vi "basic_subvi_plotPNG_v2_170407.vi"(6 "Plot and Save Options":T2={"Color"=[0, 16711680, 6618880, 16860, 16750610, 4390878, 8388847, 16775234, 5878015, 16740807], "X axis label"="example x", "Y axis label"="example y", "BG color"=16776176, "% axis off"=0.1, "% margin "=2.0, "F: JPEG\nT: PNG"=TRUE, "Font"={"Font Name"="Times New Roman", "Size"=20, "Bold"=TRUE, "Italic"=FALSE, "Underline"=FALSE, "Strikeout"=FALSE, "Color"=0}, "Plot Line Width"=2, "X format str"="%.2f", "Y format str"="%.2f", "axis range"={"Max X scale"=0.0, "Min X scale"=0.0, "Max Y scale"=0.0, "Min Y scale"=0.0}, "auto scale?"=TRUE}, 8 "Path":path, 9 "Graph ref in":refnum<vi>) -> (4 "Graph (ploted) ref out":refnum<vi>)   [LabVIEW 2020, in "BasicVIs.lvlib"]
uses:
  BasicVIs.lvlib
  <vilib>/Utility/miscctls.llb/LVFontTypeDef.ctl
panel:
  out "Graph ref in valid?":bool
  out "path out":path
  out "error out":errorcluster
  in  "error in (no error)":errorcluster
  out "Graph":cluster{dbl[], dbl[]}[](graph)=[{[0.0, 1.0, 1.0, 0.0, 0.0], [0.0, 0.0, 1.0, 1.0, 0.0]}]
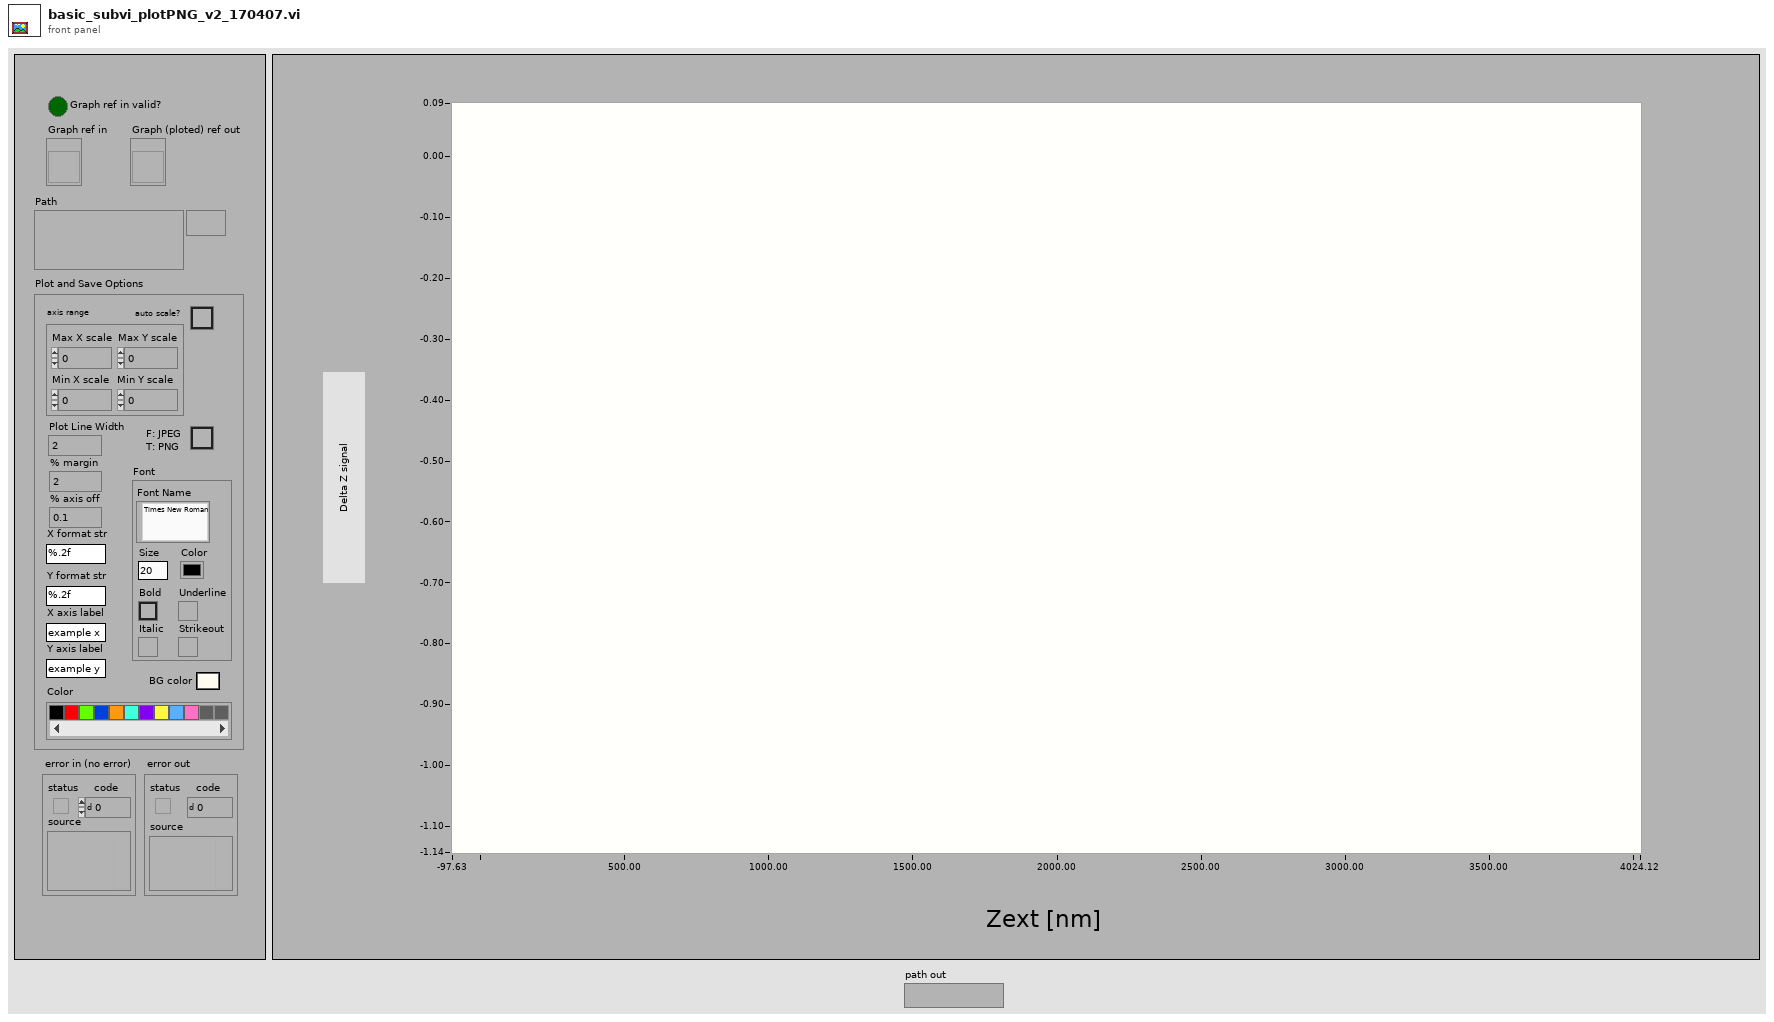
[diagram p1: front panel]
types:
  T1 = typedef "LVFontTypeDef.ctl" = cluster{"Font Name":string, "Size":u16, "Bold":bool, "Italic":bool, "Underline":bool, "Strikeout":bool, "Color":u32}
  T2 = cluster{"Color":u32[], "X axis label":string, "Y axis label":string, "BG color":u32, "% axis off":dbl, "% margin ":dbl, "F: JPEG\nT: PNG":bool, "Font":T1, "Plot Line Width":u8, "X format str":string, "Y format str":string, "axis range":cluster{"Max X scale":dbl, "Min X scale":dbl, "Max Y scale":dbl, "Min Y scale":dbl}, "auto scale?":bool}
  T3 = cluster{"Max X scale":dbl, "Min X scale":dbl, "Max Y scale":dbl, "Min Y scale":dbl}
  T4 = typedef "imagedata.ctl" = cluster{"image type":i32, "image depth":i32, "image":u8[], "mask":u8[], "colors":u32[], "Rectangle":cluster{"left":i16, "top":i16, "right":i16, "bottom":i16}}
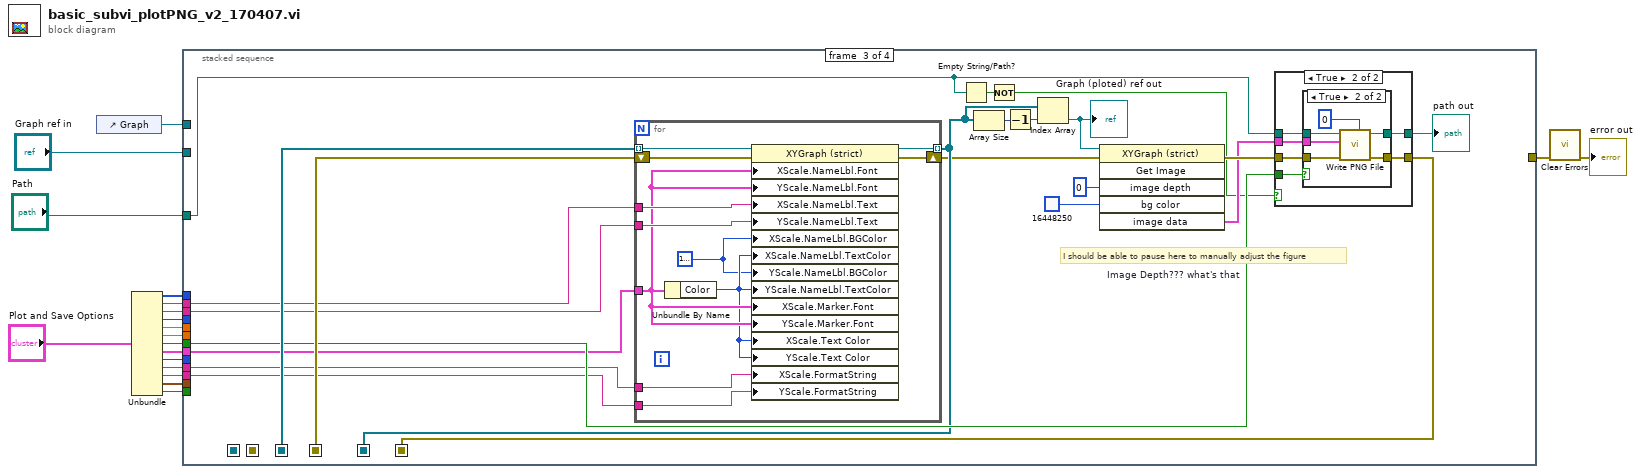
[diagram p0: block diagram]
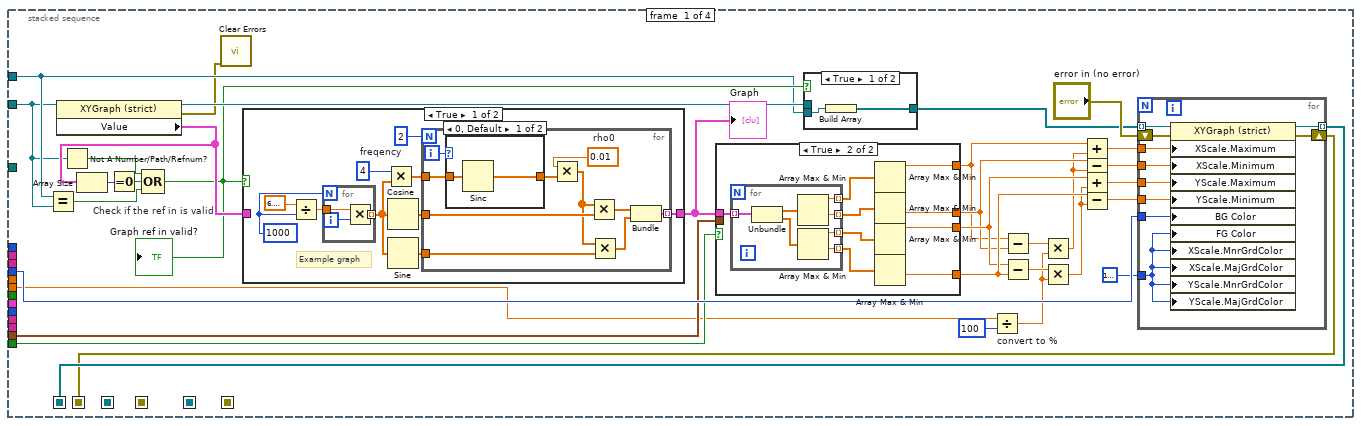
[diagram p2: hidden frame]
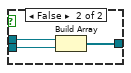
[diagram p3: hidden frame]
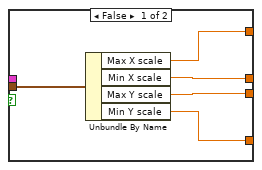
[diagram p4: hidden frame]
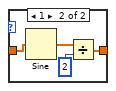
[diagram p5: hidden frame]
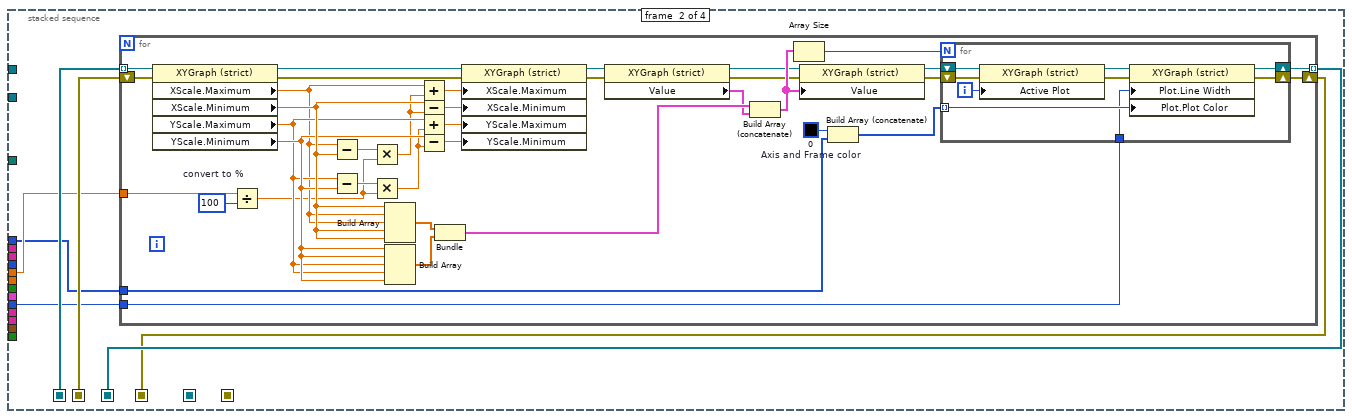
[diagram p7: hidden frame]
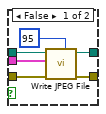
[diagram p9: hidden frame]
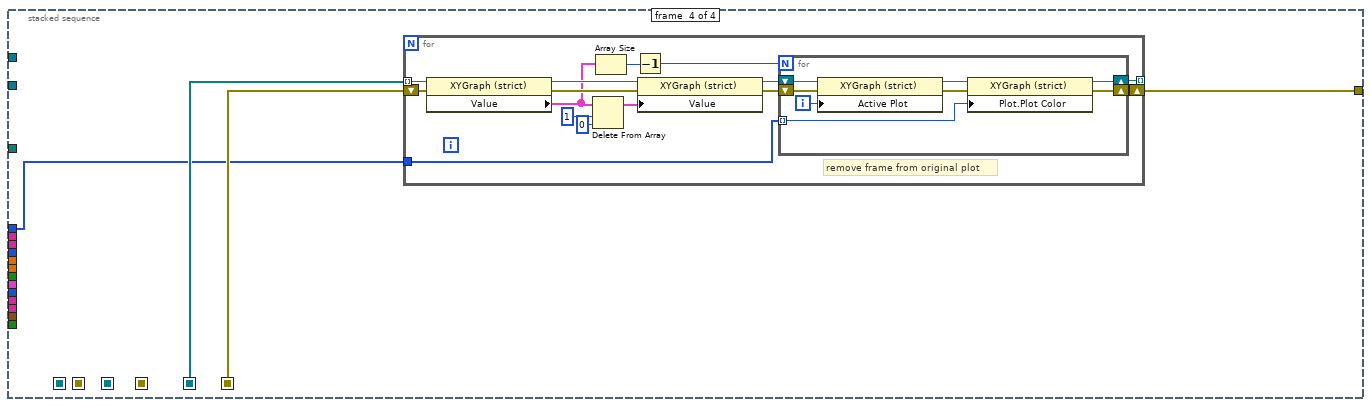
[diagram p10: hidden frame]
diagram:
  n1 = control-ref of="Graph"() -> (w8:refnum<vi>)
  n2 = Unbundle("Plot and Save Options") -> ("Color"=w3:u32[], "X axis label"=w16:string, "Y axis label"=w15:string, "BG color"=w13:u32, "% axis off"=w5:dbl, "% margin"=w4:dbl, "F: JPEG\nT: PNG"=w18:bool, "Font"=w17:T1, "Plot Line Width"=w14:u8, "X format str"=w11:string, "Y format str"=w10:string, "axis range"=w7:T3, "auto scale?"=w6:bool)
  n3 = stacked-sequence {
    seq-local: [w40 _ _ _] -> [_ w126 _ _]
    seq-local: [w33 _ _ _] -> [_ w125 _ _]
    seq-local: [_ w124 _ _] -> [_ _ w194 _]
    seq-local: [_ w122 _ _] -> [_ _ w193 _]
    seq-local: [_ _ w179 _] -> [_ _ _ w228]
    seq-local: [_ _ w177 _] -> [_ _ _ w229]
    tunnel: w4 -> [w26 _ _ _]
    tunnel: w5 -> [_ w121 _ _]
    tunnel: w3 -> [_ w120 _ w226]
    tunnel: w13 -> [w38 _ _ _]
    tunnel: w18 -> [_ _ w188 _]
    tunnel: w17 -> [_ _ w185 _]
    tunnel: w16 -> [_ _ w192 _]
    tunnel: w15 -> [_ _ w191 _]
    tunnel: "Path" -> [_ _ w173 _]
    tunnel: [_ _ _ w227] -> w2
    tunnel: w14 -> [_ w123 _ _]
    tunnel: w11 -> [_ _ w184 _]
    tunnel: w10 -> [_ _ w183 _]
    tunnel: "Graph ref in" -> [w24 _ _ _]
    tunnel: w8 -> [w31 _ _ _]
    tunnel: w7 -> [w29 _ _ _]
    tunnel: w6 -> [w30 _ _ _]
    frame #0 {
      n4 = Equal?(x=w31, y=w24) -> (x = y?=w21:bool)
      n5 = property class="XYGraph (strict)"(reference=w24) -> (reference out=w36:refnum<vi>, error out=w20:errorcluster, "Value"=w37:cluster{dbl[], dbl[]}[])  [unwired: 1 in]
      n6 = Not A Number/Path/Refnum?(number/path/refnum=w24) -> (NaN/Path/Refnum?=w23:bool)
      n7 = Array Size(array=w37) -> (size(s)=w35:i32)
      n8 = Equal To 0?(x=w35) -> (x = 0?=w22:bool)
      n9 = Compound Arithmetic op=OR "Check if the ref in is valid"(w23, w22, w21) -> (w32:bool)
      "Graph ref in valid?" <- w32
      n10 = call <vilib>:"Clear Errors.vi"("error in (no error)"=w20) -> ()  [unwired: 5 in, 2 out]
      n11 = case shown="True" w32 {
        tunnel: [w91 w119] -> w53
        tunnel: w37 -> [_ w119]
        frame True {
          w95 = 4  # freqency
          w98 = 1000
          # "Example graph"
          n12 = Divide(x=6.283185307179586, y=w98) -> (x/y=w97:dbl)
          n13 = for {
            N: w98 -> [_]
            tunnel: w97 -> [w118]
            tunnel: [w116] -> w94 mode=indexing
            i -> [w117]
            n14 = Multiply(x=w118, y=w117) -> (x*y=w116:dbl)
          }
          n15 = Multiply(x=w95, y=w94) -> (x*y=w96:dbl[])
          n16 = Cosine(x=w94) -> (cos(x)=w93:dbl[])
          n17 = Sine(x=w94) -> (sin(x)=w92:dbl[])
          n18 = for {
            N: 2 -> [_]
            tunnel: w96 -> [w109]
            tunnel: w93 -> [w107]
            tunnel: w92 -> [w105]
            tunnel: [w101] -> w91 mode=indexing
            i -> [w100]
            w103 = 0.01  # rho0
            n19 = case shown="0, Default" w100 {
              tunnel: w109 -> [w111 w115]
              tunnel: [w110 w112] -> w108
              frame 0, Default {
                n20 = Sinc(1:w111) -> (0:w110:dbl[])
              }
              frame 1 {
                n21 = Sine(x=w115) -> (sin(x)=w113:dbl[])
                n22 = Divide(x=w113, y=2) -> (x/y=w112:dbl[])
              }
            }
            n23 = Multiply(x=w103, y=w108) -> (x*y=w102:dbl[])
            n24 = Multiply(x=w102, y=w107) -> (x*y=w106:dbl[])
            n25 = Multiply(x=w102, y=w105) -> (x*y=w104:dbl[])
            n26 = Bundle(w106, w104) -> (w101:cluster{dbl[], dbl[]})  [unwired: 1 in]
          }
        }
        frame False {
        }
      }
      "Graph" <- w53
      n27 = case shown="True" w30 {
        tunnel: w53 -> [_ w72]
        tunnel: [w59 w71] -> w48
        tunnel: [w60 w70] -> w47
        tunnel: [w61 w69] -> w46
        tunnel: [w62 w68] -> w45
        tunnel: w29 -> [w63 _]
        frame False {
          n28 = Unbundle By Name(w63) -> ("Max X scale"=w62:dbl, "Min X scale"=w61:dbl, "Max Y scale"=w60:dbl, "Min Y scale"=w59:dbl)
        }
        frame True {
          n29 = for {
            tunnel: w72 -> [w79] mode=indexing
            tunnel: [w76] -> w64 mode=indexing
            tunnel: [w75] -> w65 mode=indexing
            tunnel: [w74] -> w66 mode=indexing
            tunnel: [w73] -> w67 mode=indexing
            n30 = Unbundle(w79) -> (w77:dbl[], w78:dbl[])
            n31 = Array Max & Min(array=w77) -> (max value=w76:dbl, min value=w75:dbl)  [unwired: 2 out]
            n32 = Array Max & Min(array=w78) -> (max value=w74:dbl, min value=w73:dbl)  [unwired: 2 out]
          }
          n33 = Array Max & Min(array=w64) -> (max value=w68:dbl)  [unwired: 3 out]
          n34 = Array Max & Min(array=w65) -> (min value=w69:dbl)  [unwired: 3 out]
          n35 = Array Max & Min(array=w66) -> (max value=w70:dbl)  [unwired: 3 out]
          n36 = Array Max & Min(array=w67) -> (min value=w71:dbl)  [unwired: 3 out]
        }
      }
      n37 = case shown="True" w32 {
        tunnel: [w55 w58] -> w34
        tunnel: w36 -> [_ w57]
        tunnel: w31 -> [w54 w56]
        frame True {
          n38 = Build Array(w54) -> (w55:refnum<vi>[])
        }
        frame False {
          n39 = Build Array(w57, w56) -> (w58:refnum<vi>[])
        }
      }
      n40 = Divide "convert to %"(x=w26, y=100) -> (x/y=w27:dbl)
      n41 = Subtract(x=w45, y=w46) -> (x-y=w41:dbl)
      n42 = Subtract(x=w47, y=w48) -> (x-y=w42:dbl)
      n43 = Multiply(x=w41, y=w27) -> (x*y=w43:dbl)
      n44 = Multiply(x=w42, y=w27) -> (x*y=w44:dbl)
      n45 = Add(x=w45, y=w43) -> (x+y=w49:dbl)
      n46 = Subtract(x=w46, y=w43) -> (x-y=w50:dbl)
      n47 = Add(x=w47, y=w44) -> (x+y=w51:dbl)
      n48 = Subtract(x=w48, y=w44) -> (x-y=w52:dbl)
      n49 = for {
        tunnel: w52 -> [w89]
        tunnel: w51 -> [w88]
        tunnel: w50 -> [w87]
        tunnel: w49 -> [w86]
        tunnel: [w85] -> w40 mode=indexing
        tunnel: w38 -> [w82]
        tunnel: u32 16777216 ("FG color") -> [w80]
        tunnel: w34 -> [w81] mode=indexing
        shift-right: [w84] -> w33
        shift-left: "error in (no error)" -> [w83]
        n50 = property class="XYGraph (strict)"(reference=w81, error in=w83, "XScale.Maximum"=w86, "XScale.Minimum"=w87, "YScale.Maximum"=w88, "YScale.Minimum"=w89, "BG Color"=w82, "FG Color"=w80, "XScale.MnrGrdColor"=w80, "XScale.MajGrdColor"=w80, "YScale.MnrGrdColor"=w80, "YScale.MajGrdColor"=w80) -> (reference out=w85:refnum<vi>, error out=w84:errorcluster)
      }
    }
    frame #1 {
      n51 = for {
        tunnel: w126 -> [w137] mode=indexing
        tunnel: [w135] -> w124 mode=indexing
        tunnel: w123 -> [w133]
        shift-right: [w134] -> w122
        shift-left: w125 -> [w136]
        tunnel: w121 -> [w131]
        tunnel: w120 -> [w127]
        w129 = u32 0  # Axis and Frame color
        n52 = property class="XYGraph (strict)"(reference=w137, error in=w136) -> (reference out=w156:refnum<vi>, error out=w158:errorcluster, "XScale.Maximum"=w151:dbl, "XScale.Minimum"=w155:dbl, "YScale.Maximum"=w153:dbl, "YScale.Minimum"=w154:dbl)
        n53 = Divide "convert to %"(x=w131, y=100) -> (x/y=w130:dbl)
        n54 = Subtract(x=w151, y=w155) -> (x-y=w144:dbl)
        n55 = Subtract(x=w153, y=w154) -> (x-y=w145:dbl)
        n56 = Multiply(x=w144, y=w130) -> (x*y=w150:dbl)
        n57 = Multiply(x=w145, y=w130) -> (x*y=w152:dbl)
        n58 = Build Array(w155, w151, w151, w155, w155) -> (w138:dbl[])
        n59 = Build Array(w154, w154, w153, w153, w154) -> (w139:dbl[])
        n60 = Add(x=w151, y=w150) -> (x+y=w146:dbl)
        n61 = Subtract(x=w155, y=w150) -> (x-y=w147:dbl)
        n62 = Add(x=w153, y=w152) -> (x+y=w148:dbl)
        n63 = Subtract(x=w154, y=w152) -> (x-y=w149:dbl)
        n64 = Bundle(w138, w139) -> (w143:cluster{dbl[], dbl[]})  [unwired: 1 in]
        n65 = property class="XYGraph (strict)"(reference=w156, error in=w158, "XScale.Maximum"=w146, "XScale.Minimum"=w147, "YScale.Maximum"=w148, "YScale.Minimum"=w149) -> (reference out=w157:refnum<vi>, error out=w159:errorcluster)
        n66 = property class="XYGraph (strict)"(reference=w157, error in=w159) -> (reference out=w140:refnum<vi>, error out=w141:errorcluster, "Value"=w142:cluster{dbl[], dbl[]}[])
        n67 = Build Array (concatenate)(w143, w142) -> (w160:cluster{dbl[], dbl[]}[])
        n68 = Array Size(array=w160) -> (size(s)=w163:i32)
        n69 = property class="XYGraph (strict)"(reference=w140, error in=w141, "Value"=w160) -> (reference out=w161:refnum<vi>, error out=w162:errorcluster)
        n70 = Build Array (concatenate)(w129, w127) -> (w128:u32[])
        n71 = for {
          N: w163 -> [_]
          shift-right: [w167] -> w135
          shift-left: w161 -> [w172]
          shift-right: [w166] -> w134
          shift-left: w162 -> [w171]
          tunnel: w128 -> [w165] mode=indexing
          tunnel: w133 -> [w164]
          i -> [w170]
          n72 = property class="XYGraph (strict)"(reference=w172, error in=w171, "Active Plot"=w170) -> (reference out=w169:refnum<vi>, error out=w168:errorcluster)
          n73 = property class="XYGraph (strict)"(reference=w169, error in=w168, "Plot.Line Width"=w164, "Plot.Plot Color"=w165) -> (reference out=w167:refnum<vi>, error out=w166:errorcluster)
        }
      }
    }
    frame #2 {
      w187 = 0  # Image Depth??? what's that
      # "I should be able to pause here to manually adjust the figure"
      n74 = for {
        tunnel: w194 -> [w225] mode=indexing
        tunnel: w192 -> [w223]
        tunnel: w191 -> [w222]
        tunnel: [w221] -> w179 mode=indexing
        tunnel: w185 -> [w220]
        shift-right: [w218] -> w178
        shift-left: w193 -> [w224]
        tunnel: w184 -> [w217]
        tunnel: w183 -> [w216]
        w215 = u32 16777216 ("FG color")
        n75 = Unbundle By Name(w220) -> ("Color"=w219:u32)
        n76 = property class="XYGraph (strict)"(reference=w225, error in=w224, "XScale.NameLbl.Font"=w220, "YScale.NameLbl.Font"=w220, "XScale.NameLbl.Text"=w223, "YScale.NameLbl.Text"=w222, "XScale.NameLbl.BGColor"=w215, "XScale.NameLbl.TextColor"=w219, "YScale.NameLbl.BGColor"=w215, "YScale.NameLbl.TextColor"=w219, "XScale.Marker.Font"=w220, "YScale.Marker.Font"=w220, "XScale.Text Color"=w219, "YScale.Text Color"=w219, "XScale.FormatString"=w217, "YScale.FormatString"=w216) -> (reference out=w221:refnum<vi>, error out=w218:errorcluster)
      }
      n77 = Empty String/Path?(string/path=w173) -> (empty?=w175:bool)
      n78 = Array Size(array=w179) -> (size(s)=w182:i32)
      n79 = Not(x=w175) -> (.not. x?=w174:bool)
      n80 = Decrement(x=w182) -> (x-1=w181:i32)
      n81 = Index Array(array=w179, index=w181) -> (element=w180:refnum<vi>)
      "Graph (ploted) ref out" <- w180
      n82 = invoke class="XYGraph (strict)" method="Get Image"(reference=w180, error in=w178, "image depth"=w187, "bg color"=u32 16448250 ("FG color")) -> (error out=w190:errorcluster, "image data"=w189:T4)  [unwired: 2 in, 4 out]
      n83 = case shown="True" w174 {
        tunnel: w190 -> [w195 w202]
        tunnel: w189 -> [_ w201]
        tunnel: w188 -> [_ w200]
        tunnel: w173 -> [w196 w199]
        tunnel: [w195 w198] -> w177
        tunnel: [w196 w197] -> w176
        frame False {
        }
        frame True {
          n84 = case shown="True" w200 {
            tunnel: w201 -> [w207 w214]
            tunnel: w199 -> [w208 w213]
            tunnel: w202 -> [w206 w212]
            tunnel: [w204 w210] -> w198
            tunnel: [w203 w209] -> w197
            frame False {
              n85 = call <vilib>:"Write JPEG File.vi"("quality (80)"=95, "error in (no error)"=w206, "image data"=w207, "path to JPEG file"=w208) -> ("error out"=w204:errorcluster, "path"=w203:path)  [unwired: 6 in]
            }
            frame True {
              n86 = call <vilib>:"Write PNG File.vi"("compression (default)"=0, "error in (no error)"=w212, "image data"=w214, "path to PNG file"=w213) -> ("error out"=w210:errorcluster, "path"=w209:path)  [unwired: 6 in]
            }
          }
        }
      }
      "path out" <- w176
    }
    frame #3 {
      n87 = for {
        shift-right: [w237] -> w227
        shift-left: w229 -> [w240]
        tunnel: w228 -> [w239] mode=indexing
        tunnel: [w238] -> _ mode=indexing
        tunnel: w226 -> [w233]
        # "remove frame from original plot"
        n88 = property class="XYGraph (strict)"(reference=w239, error in=w240) -> (reference out=w244:refnum<vi>, error out=w243:errorcluster, "Value"=w236:cluster{dbl[], dbl[]}[])
        n89 = Delete From Array(array=w236, length=1, index=0) -> (array with subset deleted=w232:cluster{dbl[], dbl[]}[])  [unwired: 1 out]
        n90 = Array Size(array=w236) -> (size(s)=w234:i32)
        n91 = Decrement(x=w234) -> (x-1=w231:i32)
        n92 = property class="XYGraph (strict)"(reference=w244, error in=w243, "Value"=w232) -> (reference out=w242:refnum<vi>, error out=w241:errorcluster)
        n93 = for {
          N: w231 -> [_]
          shift-right: [w247] -> w238
          shift-left: w242 -> [w252]
          shift-right: [w246] -> w237
          shift-left: w241 -> [w251]
          tunnel: w233 -> [w245] mode=indexing
          i -> [w250]
          n94 = property class="XYGraph (strict)"(reference=w252, error in=w251, "Active Plot"=w250) -> (reference out=w249:refnum<vi>, error out=w248:errorcluster)
          n95 = property class="XYGraph (strict)"(reference=w249, error in=w248, "Plot.Plot Color"=w245) -> (reference out=w247:refnum<vi>, error out=w246:errorcluster)
        }
      }
    }
  }
  n96 = call <vilib>:"Clear Errors.vi"("error in (no error)"=w2) -> ("error out"=→"error out":errorcluster)  [unwired: 5 in, 1 out]
